vi "basic read one field.vi"() -> (2 "Field":dbl[unit])   [LabVIEW 2012]
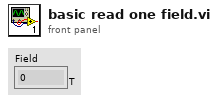
[diagram p1: front panel]
types:
  T1 = cluster{"function (0:volts DC)":u16, "range (0:auto)":u16, "rate (0:slow)":u16, "trigger mode (0:internal)":u16, "Autorange":bool}
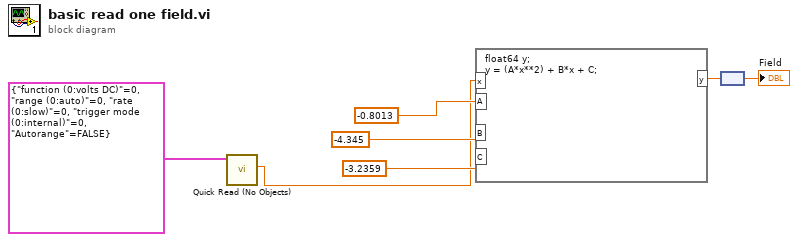
[diagram p0: block diagram]
diagram:
  n1 = call "Quick Read (No Objects).vi"("Fluke Multimeter In"=T1 {"function (0:volts DC)"=0, "range (0:auto)"=0, "rate (0:slow)"=0, "trigger mode (0:internal)"=0, "Autorange"=FALSE}) -> ("measurement"=w1:dbl)  [unwired: 7 in, 3 out]
  n2 = formula code="float64 y;\ny = (A*x**2) + B*x + C;"("x"=w1, "A"=-0.8013, "B"=-4.345, "C"=-3.2359) -> ("y"=w2:dbl)
  n3 = node(w2) -> (→"Field":dbl[unit])
